vi "ke37xx Detect Channel Match.vi"(8 "error in (no error)":errorcluster, 9 "Reset Matching Latch After Detection (False)":bool, 10 "Channel to Check for Match":string, 11 "VISA Resource Name":refnum<visa-resource-name>) -> (0 "error out":errorcluster, 2 "Matched":bool, 3 "VISA Resource Name Out":refnum<visa-resource-name>)   [LabVIEW 2009, in "Keithley 3700 Series.lvlib"]
doc: "This VI determines if the specified channel has detected a match condition."
uses:
  <instrlib>/Keithley 3706/Keithley 3700 Series.lvlib
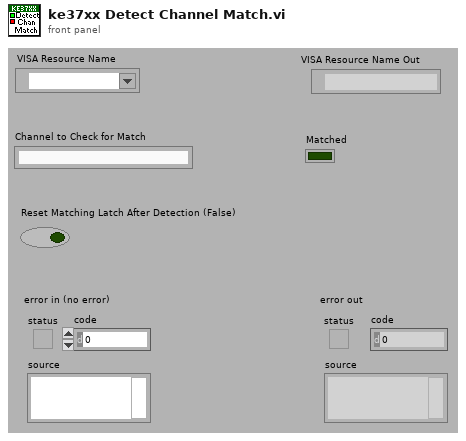
[diagram p1: front panel]
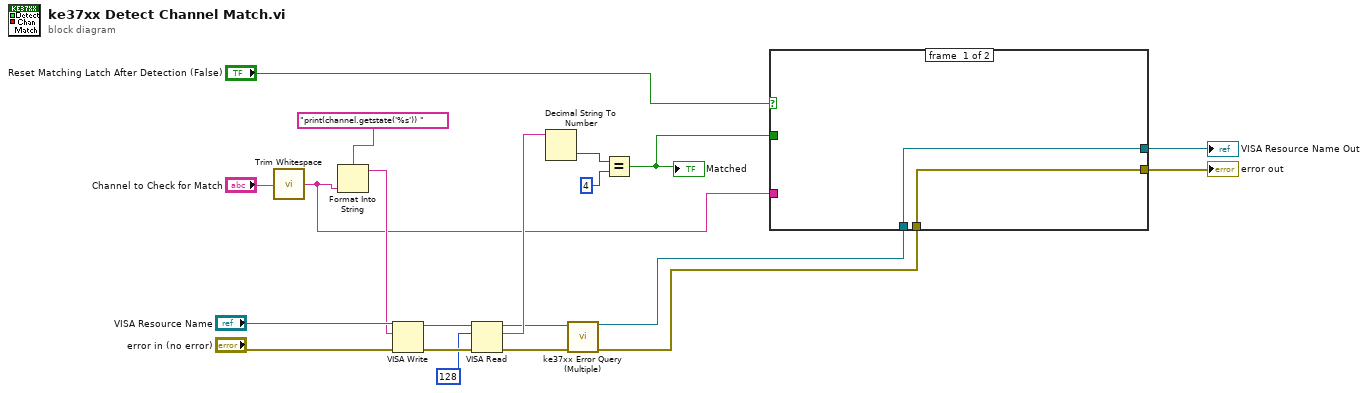
[diagram p0: block diagram]
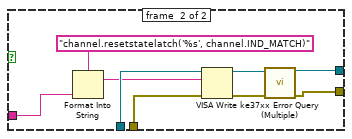
[diagram p3: hidden frame]
diagram:
  n1 = call <vilib>:"Trim Whitespace.vi"("string"="Channel to Check for Match") -> ("trimmed string"=w7:string)  [unwired: 1 in]
  n2 = Format Into String(format string="print(channel.getstate('%s')) ", w7) -> (resulting string=w17:string)  [unwired: 2 in, 1 out]
  n3 = VISA Write(VISA resource name="VISA Resource Name", write buffer=w17, error in (no error)="error in (no error)") -> (VISA resource name out=w15:refnum<visa-resource-name>, error out=w16:errorcluster)  [unwired: 1 out]
  n4 = VISA Read(VISA resource name=w15, byte count=128, error in (no error)=w16) -> (VISA resource name out=w6:refnum<visa-resource-name>, read buffer=w12:string, error out=w5:errorcluster)  [unwired: 1 out]
  n5 = Decimal String To Number(string=w12) -> (number=w11:i32)  [unwired: 3 out]
  n6 = call <instrlib>:"ke37xx Error Query (Multiple).vi"("VISA resource name"=w6, "error in (no error)"=w5) -> ("VISA resource name out"=w4:refnum<visa-resource-name>, "error out"=w3:errorcluster)  [unwired: 12 out]
  n7 = Equal?(x=w11, y=4) -> (x = y?=w8:bool)
  "Matched" <- w8
  n8 = case shown="True" "Reset Matching Latch After Detection (False)" {
    tunnel: w8 -> [_ w28]
    tunnel: w7 -> [_ w27]
    tunnel: w4 -> [w21 w26]
    tunnel: w3 -> [w22 w25]
    tunnel: [w22 w24] -> w2
    tunnel: [w21 w23] -> w1
    frame #0 {
    }
    frame #1 {
      n9 = case shown="False" w28 {
        tunnel: w27 -> [_ w38]
        tunnel: w26 -> [w29 w35]
        tunnel: w25 -> [w30 w34]
        tunnel: [w30 w33] -> w24
        tunnel: [w29 w32] -> w23
        frame #0 {
        }
        frame #1 {
          n10 = Format Into String(format string="channel.resetstatelatch('%s', channel.IND_MATCH)", w38) -> (resulting string=w31:string)  [unwired: 2 in, 1 out]
          n11 = VISA Write(VISA resource name=w35, write buffer=w31, error in (no error)=w34) -> (VISA resource name out=w37:refnum<visa-resource-name>, error out=w36:errorcluster)  [unwired: 1 out]
          n12 = call <instrlib>:"ke37xx Error Query (Multiple).vi"("VISA resource name"=w37, "error in (no error)"=w36) -> ("VISA resource name out"=w32:refnum<visa-resource-name>, "error out"=w33:errorcluster)  [unwired: 12 out]
        }
      }
    }
  }
  "VISA Resource Name Out" <- w1
  "error out" <- w2
